vi "Encode.vi"(8 "error in":errorcluster, 10 "all rows":string[][](array[string]), 11 "file path (dialog if empty)":path) -> (0 "error out":errorcluster, 2 "Encoded Data":string, 3 "file path (dialog if empty) 2":path)   [LabVIEW 2022 SP3]
uses:
  <vilib>/Utility/file.llb/Write Delimited Spreadsheet (string).vi
panel:
  # "ENCODE"
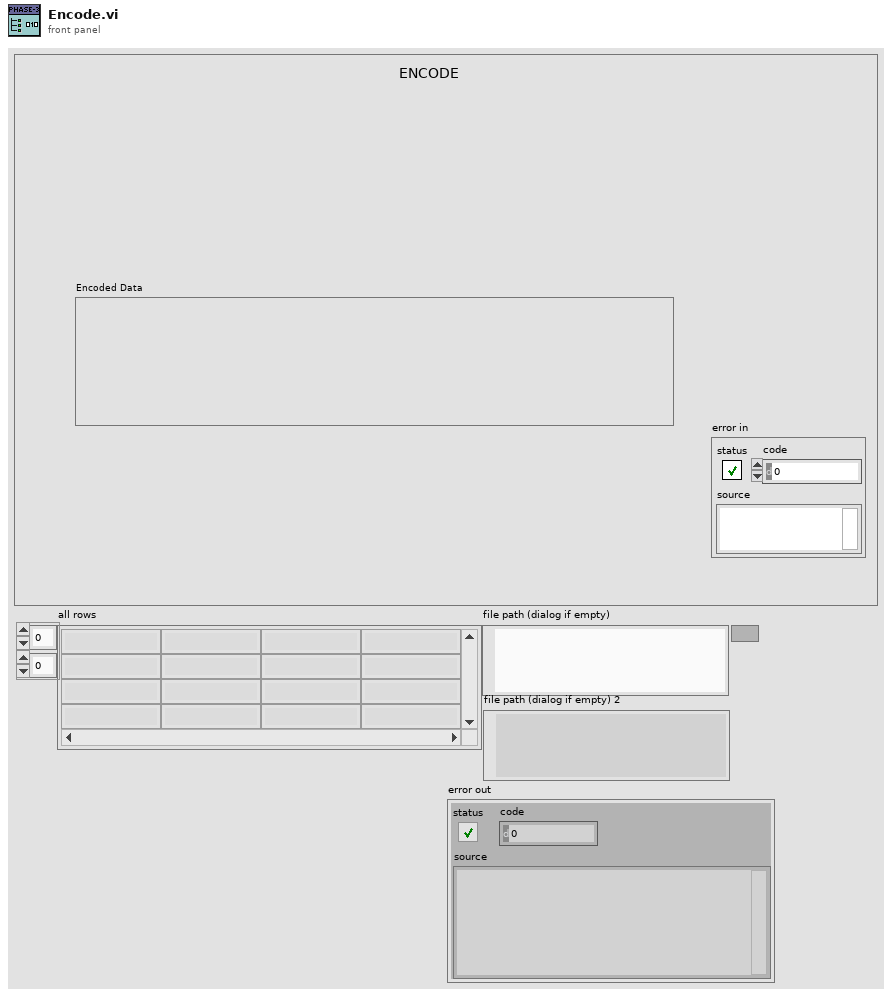
[diagram p1: front panel]
types:
  T1 = cluster{"unsigned byte array[0]":u8, "unsigned byte array[1]":u8, "unsigned byte array[2]":u8}
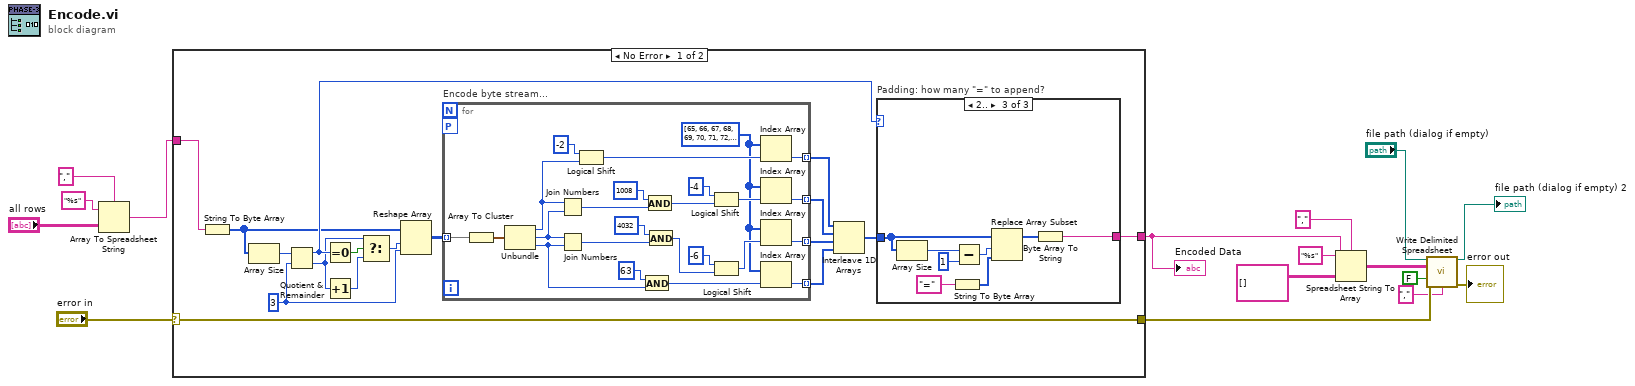
[diagram p0: block diagram]
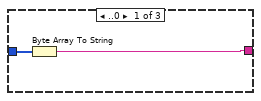
[diagram p2: hidden frame]
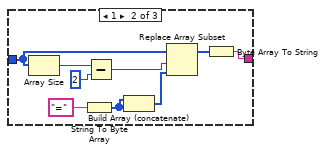
[diagram p3: hidden frame]
diagram:
  n1 = Array To Spreadsheet String(delimiter (Tab)=",", array="all rows", 3:"%s" ("format string")) -> (spreadsheet string=w5:string)
  n2 = case shown="No Error" "error in" {
    selector: "error in" -> [w18 w78]
    tunnel: [w18 w78] -> w14
    tunnel: [w20 w77] -> w15
    tunnel: w5 -> [w17 w77]
    frame No Error {
      w23 = 3 ("y")
      n3 = String To Byte Array(string=w17) -> (unsigned byte array=w24:u8[])
      n4 = Array Size(array=w24) -> (size(s)=w19:i32)
      n5 = Quotient & Remainder(x=w19, y=w23) -> (x-y*floor(x/y)=w32:i32, floor(x/y)=w26:i32)
      n6 = Equal To 0?(x=w32) -> (x = 0?=w33:bool)
      n7 = Increment(x=w26) -> (x+1=w27:i32)
      n8 = Select(t=w26, s=w33, f=w27) -> (s? t:f=w22:i32)
      n9 = Reshape Array(w24, w22, w23) -> (w21:u8[][])
      n10 = for "Encode byte stream..." {
        tunnel: [w36] -> w28 mode=indexing
        tunnel: [w37] -> w29 mode=indexing
        tunnel: [w38] -> w30 mode=indexing
        tunnel: [w39] -> w31 mode=indexing
        workers-P: _ -> [_]
        tunnel: w21 -> [w34] mode=indexing
        w35 = u8[] [65, 66, 67, 68, 69, 70, 71, 72, 73, 74, 75, 76, 77, 78, 79, 80, 81, 82, 83, 84, 85, 86, 87, 88, 89, 90, 97, 98, 99, 100, 101, 102, 103, 104, 105, 106, 107, 108, 109, 110, 111, 112, 113, 114, 115, 116, 117, 118, 119, 120, 121, 122, 48, 49, 50, 51, 52, 53, 54, 55, 56, 57, 43, 47] ("unsigned byte array")
        n11 = Array To Cluster(array=w34) -> (cluster=w57:T1)
        n12 = Unbundle(w57) -> ("unsigned byte array[0]"=w46:u8, "unsigned byte array[1]"=w51:u8, "unsigned byte array[2]"=w45:u8)
        n13 = Join Numbers(hi=w46, lo=w51) -> ((hi.lo)=w55:u16)
        n14 = Join Numbers(hi=w51, lo=w45) -> ((hi.lo)=w50:u16)
        n15 = Logical Shift(y=i8 -2, x=w46) -> (x << y=w43:u8)
        n16 = And(x=u8 63, y=w45) -> (x .and. y?=w40:u8)
        n17 = And(x=u16 1008, y=w55) -> (x .and. y?=w53:u16)
        n18 = And(x=u16 4032, y=w50) -> (x .and. y?=w48:u16)
        n19 = Logical Shift(y=i8 -4, x=w53) -> (x << y=w42:u16)
        n20 = Logical Shift(y=i8 -6, x=w48) -> (x << y=w41:u16)
        n21 = Index Array(array=w35, index=w43) -> (element=w39:u8)
        n22 = Index Array(array=w35, index=w42) -> (element=w38:u8)
        n23 = Index Array(array=w35, index=w41) -> (element=w37:u8)
        n24 = Index Array(array=w35, index=w40) -> (element=w36:u8)
      }
      n25 = Interleave 1D Arrays(w31, w30, w29, w28) -> (w25:u8[])
      n26 = case "Padding: how many \"=\" to append?" shown="2.." w32 {
        tunnel: [w58 w65 w73] -> w20
        tunnel: w25 -> [w59 w63 w71]
        frame ..0 {
          n27 = Byte Array To String(unsigned byte array=w59) -> (string=w58:string)
        }
        frame 1 {
          n28 = Array Size(array=w63) -> (size(s)=w64:i32)
          n29 = String To Byte Array(string="=") -> (unsigned byte array=w61:u8[])
          n30 = Subtract(x=w64, y=2) -> (x-y=w67:i32)
          n31 = Build Array (concatenate)(w61, w61) -> (w60:u8[])
          n32 = Replace Array Subset(array=w63, new element=w60, index=w67) -> (w66:u8[])
          n33 = Byte Array To String(unsigned byte array=w66) -> (string=w65:string)
        }
        frame 2.. {
          n34 = Array Size(array=w71) -> (size(s)=w72:i32)
          n35 = String To Byte Array(string="=") -> (unsigned byte array=w69:u8[])
          n36 = Subtract(x=w72, y=1) -> (x-y=w75:i32)
          n37 = Replace Array Subset(array=w71, new element=w69, index=w75) -> (w74:u8[])
          n38 = Byte Array To String(unsigned byte array=w74) -> (string=w73:string)
        }
      }
    }
    frame Error {
    }
  }
  "Encoded Data" <- w15
  n39 = Spreadsheet String To Array(delimiter (Tab)=",", format string="%s", spreadsheet string=w15, array type (2D Dbl)=string[][] [] ("all rows")) -> (array=w11:string[][])
  n40 = call-poly <vilib>:"Write Delimited Spreadsheet.vi"("file path (dialog if empty)"="file path (dialog if empty)", "2D data"=w11, "append to file? (new file:F)"=FALSE, "error in (no error)"=w14, "delimiter (\\t)"="," ("delimiter (\\t)")) -> ("new file path (Not A Path if cancelled)"=→"file path (dialog if empty) 2":path, "error out"=→"error out":errorcluster)  [unwired: 9 in]
